vi "Write TreeBar.vi"(8 "error in (no error)":errorcluster, 10 "Event Sequencer.lvlib:BetterTreeBar.lvclass":refnum<class "BetterHorizontalBar.lvclass">, 11 "BetterHandle in":refnum<class "BetterHandle.lvclass">) -> (0 "error out":errorcluster, 3 "BetterHandle out":refnum<class "BetterHandle.lvclass">)   [LabVIEW 2020, in "BetterDragAndDrop.lvlib" / "BetterHandle.lvclass"]
uses:
  BetterHandle.lvclass
  BetterTreeBar/BetterHorizontalBar.lvclass
  BetterHandle.lvclass/BetterHandle.ctl
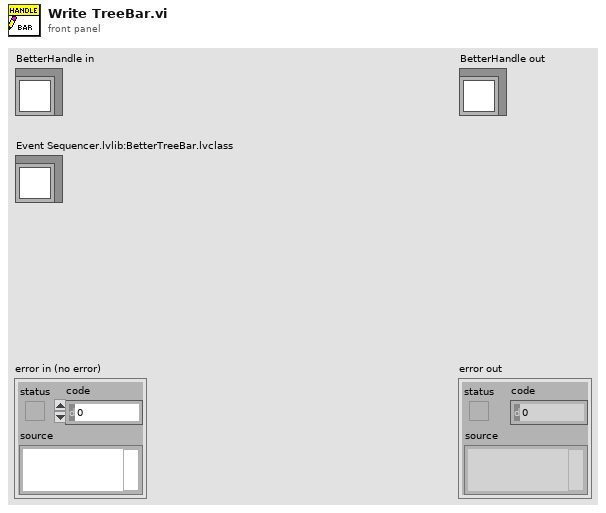
[diagram p1: front panel]
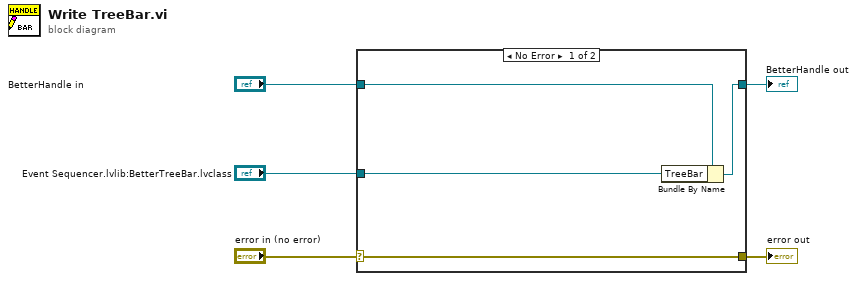
[diagram p0: block diagram]
diagram:
  n1 = case shown="No Error" "error in (no error)" {
    selector: "error in (no error)" -> [w9 w10]
    tunnel: [w9 w10] -> w4
    tunnel: [w7 w11] -> w2
    tunnel: "BetterHandle in" -> [w8 w11]
    tunnel: "Event Sequencer.lvlib:BetterTreeBar.lvclass" -> [w6 _]
    frame No Error {
      n2 = Bundle By Name(cluster=w8, "TreeBar"=w6) -> (w7:refnum<class "BetterHandle.lvclass">)
    }
    frame Error {
    }
  }
  "error out" <- w4
  "BetterHandle out" <- w2
